vi "SwerveOdometry_UpdateWithTimeX.vi"(7 "SWERVE_DRIVE_KINEMATICS":T1 {"PrevCoR"."Y" format="%14.3f"; "PrevCoR"."X" format="%14.3f"; "Modules"."Y" format="%14.3f"; "Modules"."X" format="%14.3f"}, 8 "gyroAngle":T5={"VALUE"=0.0, "COS"=1.0, "SIN"=0.0} {"SIN" format="%13.4f"; "COS" format="%13.4f"; "VALUE" format="%13.4f"}, 9 "module States":T4[](array[typedef]) {"Angle"."SIN" format="%13.4f"; "Angle"."COS" format="%13.4f"; "Angle"."VALUE" format="%13.4f"}, 10 "Time":dbl, 11 "in SWERVE_DRIVE_ODOMETRY":T7={"POSE"={"TRANSLATION"={"X"=0.0, "Y"=0.0}, "ROTATION"={"VALUE"=0.0, "COS"=1.0, "SIN"=0.0}}, "GyroOffset"={"VALUE"=0.0, "COS"=1.0, "SIN"=0.0}, "PreviousAngle"={"VALUE"=0.0, "COS"=1.0, "SIN"=0.0}, "PrevTime"=0.0} {"PreviousAngle"."SIN" format="%13.4f"; "PreviousAngle"."COS" format="%13.4f"; "PreviousAngle"."VALUE" format="%13.4f"; "GyroOffset"."SIN" format="%13.4f"; "GyroOffset"."COS" format="%13.4f"; "GyroOffset"."VALUE" format="%13.4f"; "POSE"."ROTATION"."SIN" format="%13.4f"; "POSE"."ROTATION"."COS" format="%13.4f"; "POSE"."ROTATION"."VALUE" format="%13.4f"; "POSE"."TRANSLATION"."Y" format="%14.3f"; "POSE"."TRANSLATION"."X" format="%14.3f"}) -> (1 "robot POSE":T6={"TRANSLATION"={"X"=0.0, "Y"=0.0}, "ROTATION"={"VALUE"=0.0, "COS"=1.0, "SIN"=0.0}} {"ROTATION"."SIN" format="%13.4f"; "ROTATION"."COS" format="%13.4f"; "ROTATION"."VALUE" format="%13.4f"; "TRANSLATION"."Y" format="%14.3f"; "TRANSLATION"."X" format="%14.3f"}, 3 "out SWERVE_DRIVE_ODOMETRY":T7={"POSE"={"TRANSLATION"={"X"=0.0, "Y"=0.0}, "ROTATION"={"VALUE"=0.0, "COS"=1.0, "SIN"=0.0}}, "GyroOffset"={"VALUE"=0.0, "COS"=1.0, "SIN"=0.0}, "PreviousAngle"={"VALUE"=0.0, "COS"=1.0, "SIN"=0.0}, "PrevTime"=0.0} {"PreviousAngle"."SIN" format="%13.4f"; "PreviousAngle"."COS" format="%13.4f"; "PreviousAngle"."VALUE" format="%13.4f"; "GyroOffset"."SIN" format="%13.4f"; "GyroOffset"."COS" format="%13.4f"; "GyroOffset"."VALUE" format="%13.4f"; "POSE"."ROTATION"."SIN" format="%13.4f"; "POSE"."ROTATION"."COS" format="%13.4f"; "POSE"."ROTATION"."VALUE" format="%13.4f"; "POSE"."TRANSLATION"."Y" format="%14.3f"; "POSE"."TRANSLATION"."X" format="%14.3f"})   [LabVIEW 2019, in "Trajectory_Library.lvlib"]
doc: "Updates the robot's position on the field using forward kinematics and integration of the pose over time. This method takes in the current time as a parameter to calculate period (difference between two timestamps). The period is used to calculate the change in distance from a velocity. Thisalso takes in an angle parameter which is used instead of the angular rate that is calculated from forward kinematics.\n\nParameters:\n - InSwerveDriveOdometry - This data structure \n - currentTime - The current time in seconds.\n - gyroAngle - The angle reported by the gyroscope.\n - moduleStates - The current state of all swerve modules. Please provide the states in the same order in which you instantiated your SwerveDriveKinematics.\n\nReturns:\n - OutSwerveDriveOdometry - Updated data structure\n - The new pose of the robot."
uses:
  Trajectory_Library.lvlib
  ROTATION2D.ctl
  SWERVE_DRIVE_ODOMETRY.ctl
  POSE2D.ctl
  TRANSLATION2D.ctl
  SWERVE_DRIVE_MODULE_STATE.ctl
  SWERVE_DRIVE_KINEMATICS.ctl
  <vilib>/Analysis/Matrix/Datatypes/RealMatrix.ctl
  Rotation_RotateBy.vi
  Rotation_UnaryMinus.vi
  Rotation_CreateXY.vi
  Rotation_CreateAngle.vi
  Util_CalcDist.vi
  <vilib>/Analysis/Matrix/NI_Matrix.lvlib
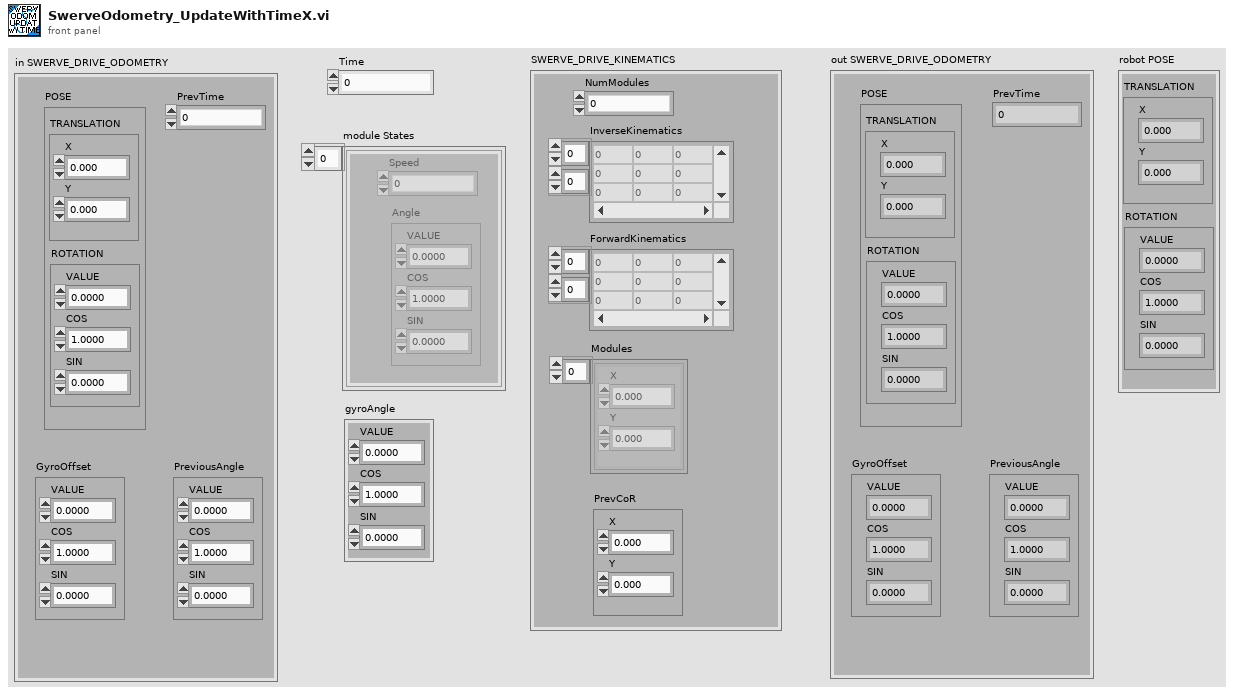
[diagram p1: front panel]
types:
  T1 = typedef "Trajectory_Library.lvlib/SWERVE_DRIVE_KINEMATICS.ctl" = cluster{"NumModules":i32, "InverseKinematics":T2, "ForwardKinematics":T2, "Modules":T3[], "PrevCoR":T3}
  T2 = typedef "NI_Matrix.lvlib/RealMatrix.ctl" = dbl[][]
  T3 = typedef "Trajectory_Library.lvlib/TRANSLATION2D.ctl" = cluster{"X":dbl, "Y":dbl}
  T4 = typedef "Trajectory_Library.lvlib/SWERVE_DRIVE_MODULE_STATE.ctl" = cluster{"Speed":dbl, "Angle":T5}
  T5 = typedef "Trajectory_Library.lvlib/ROTATION2D.ctl" = cluster{"VALUE":dbl, "COS":dbl, "SIN":dbl}
  T6 = typedef "Trajectory_Library.lvlib/POSE2D.ctl" = cluster{"TRANSLATION":T3, "ROTATION":T5}
  T7 = typedef "Trajectory_Library.lvlib/SWERVE_DRIVE_ODOMETRY.ctl" = cluster{"POSE":T6, "GyroOffset":T5, "PreviousAngle":T5, "PrevTime":dbl}
  T8 = typedef "Trajectory_Library.lvlib/CHASSIS_SPEEDS.ctl" = cluster{"vX":dbl, "vY":dbl, "vOmega":dbl}
  T9 = typedef "Trajectory_Library.lvlib/TWIST2D.ctl" = cluster{"dX":dbl, "dY":dbl, "dTHETA":dbl}
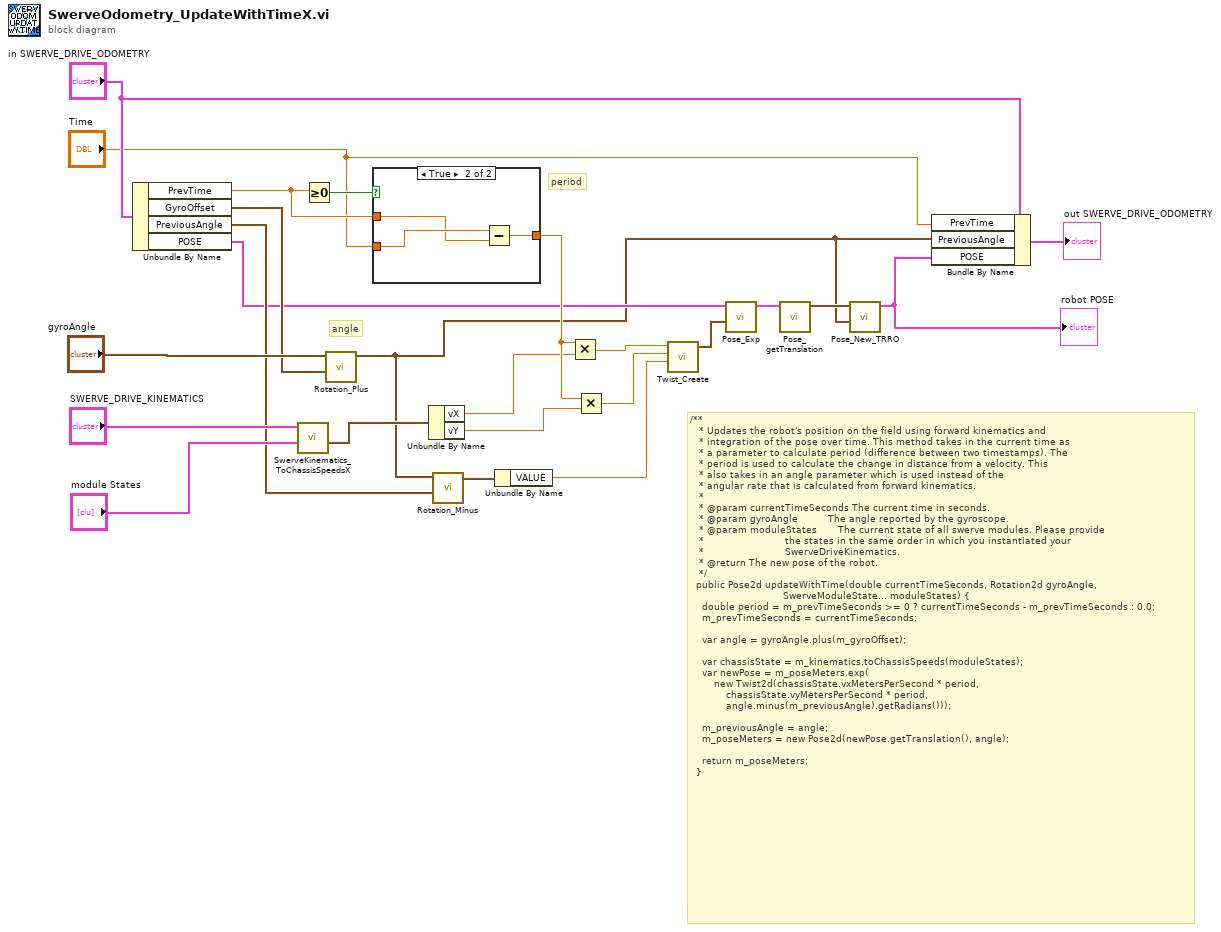
[diagram p0: block diagram]
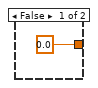
[diagram p2: hidden frame]
diagram:
  # "angle"
  # "period"
  # "/**\n   * Updates the robot's position on the field using forward kinematics and\n   * integration of the pose over time. This method takes in the current time as\n   * a parameter to calculate period (difference between two timestamps). The\n   * period is used to calculate the change in distance from a velocity. This\n   * also takes in an angle parameter which is used instead of the\n   * angular rate that is calculated from forward kinematics.\n   *\n   * @param currentTimeSeconds The current time in seconds.\n   * @param gyroAngle          The angle reported by the gyroscope.\n   * @param moduleStates       The current state of all swerve modules. Please provide\n   *                           the states in the same order in which you instantiated your\n   *                           SwerveDriveKinematics.\n   * @return The new pose of the robot.\n   */\n  public Pose2d updateWithTime(double currentTimeSeconds, Rotation2d gyroAngle,\n                               SwerveModuleState... moduleStates) {\n    double period = m_prevTimeSeconds >= 0 ? currentTimeSeconds - m_prevTimeSeconds : 0.0;\n    m_prevTimeSeconds = currentTimeSeconds;\n\n    var angle = gyroAngle.plus(m_gyroOffset);\n\n    var chassisState = m_kinematics.toChassisSpeeds(moduleStates);\n    var newPose = m_poseMeters.exp(\n        new Twist2d(chassisState.vxMetersPerSecond * period,\n            chassisState.vyMetersPerSecond * period,\n            angle.minus(m_previousAngle).getRadians()));\n\n    m_previousAngle = angle;\n    m_poseMeters = new Pose2d(newPose.getTranslation(), angle);\n\n    return m_poseMeters;\n  }"
  n1 = Unbundle By Name("in SWERVE_DRIVE_ODOMETRY") -> ("PrevTime"=w21:dbl, "GyroOffset"=w18:T5, "PreviousAngle"=w9:T5, "POSE"=w6:T6)
  n2 = call "SwerveKinematics_ToChassisSpeedsX.vi"("WheelStates"="module States", "in SWERVE_DRIVE_KINEMATICS"="SWERVE_DRIVE_KINEMATICS") -> ("Chassis Speed"=w15:T8)  [unwired: 9 in]
  n3 = Greater Or Equal To 0?(x=w21) -> (x >= 0?=w22:bool)
  n4 = call "Rotation_Plus.vi"("other ROTATION"=w18, "in ROTATION"="gyroAngle") -> ("out ROTATION"=w2:T5)  [unwired: 9 in]
  n5 = case shown="True" w22 {
    tunnel: "Time" -> [_ w28]
    tunnel: w21 -> [_ w27]
    tunnel: [0.0 w26] -> w14
    frame False {
    }
    frame True {
      n6 = Subtract(x=w28, y=w27) -> (x-y=w26:dbl)
    }
  }
  n7 = Unbundle By Name(w15) -> ("vX"=w13:dbl, "vY"=w12:dbl)
  n8 = call "Rotation_Minus.vi"("other ROTATION"=w9, "in ROTATION"=w2) -> ("out ROTATION"=w8:T5)  [unwired: 9 in]
  n9 = Unbundle By Name(w8) -> ("VALUE"=w7:dbl)
  n10 = Multiply(x=w14, y=w13) -> (x*y=w11:dbl)
  n11 = Multiply(x=w14, y=w12) -> (x*y=w10:dbl)
  n12 = call "Twist_Create.vi"("dTHETA"=w7, "dY"=w10, "dX"=w11) -> ("TWIST"=w5:T9)  [unwired: 8 in]
  n13 = call "Pose_Exp.vi"("TWIST"=w5, "POSE"=w6) -> ("UpdatedPose"=w4:T6)  [unwired: 9 in]
  n14 = call "Pose_getTranslation.vi"("in POSE"=w4) -> ("outTRANSLATION"=w3:T3)  [unwired: 10 in]
  n15 = call "Pose_New_TRRO.vi"("ROTATION"=w2, "TRANSLATION"=w3) -> ("outPOSE"=w1:T6)  [unwired: 9 in]
  "robot POSE" <- w1
  n16 = Bundle By Name(cluster="in SWERVE_DRIVE_ODOMETRY", "PrevTime"="Time", "PreviousAngle"=w2, "POSE"=w1) -> (→"out SWERVE_DRIVE_ODOMETRY":T7)
